vi "Test.vi"() -> ()   [LabVIEW 2011]
panel:
  out "数值":i32
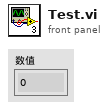
[diagram p1: front panel]
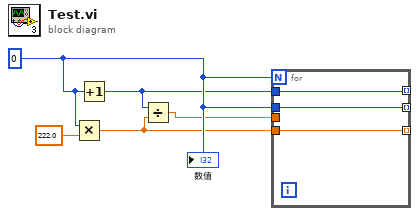
[diagram p0: block diagram]
diagram:
  w5 = 0
  n1 = Multiply(x=w5, y=222.0) -> (x*y=w2:dbl)
  n2 = Increment(x=w5) -> (x+1=w3:i32)
  n3 = Divide(x=w3, y=w2) -> (x/y=w1:dbl)
  n4 = for {
    N: w5 -> [_]
    tunnel: w5 -> [w8]
    tunnel: w3 -> [w6]
    tunnel: w2 -> [w7]
    tunnel: [w8] -> _ mode=indexing
    tunnel: [w7] -> _ mode=indexing
    tunnel: [w6] -> _ mode=indexing
    tunnel: w1 -> [_]
  }
  "数值" <- w5
